vi "Enqueue.vi"(0 "Queue Ref In":refnum<queue>, 5 "State In":string, 11 "error in (no error)":errorcluster) -> (4 "Queue Ref Out":refnum<queue>, 15 "error out":errorcluster)   [LabVIEW 2019, in "Queue Driver.lvlib"]
uses:
  Queue Driver.lvlib
  TypeDefs/Queue Data.ctl
  TypeDefs/Queue Operation.ctl
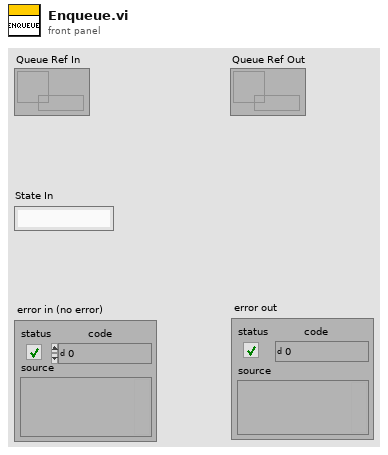
[diagram p1: front panel]
types:
  T1 = typedef "Queue Driver.lvlib/Queue Operation.ctl" = enum16{"Create", "Enqueue", "EnqueueN", "Dequeue", "Flush", "Destroy"}
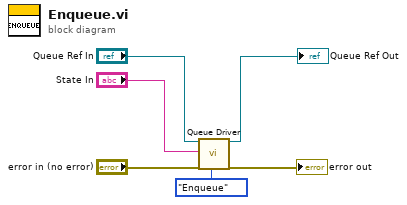
[diagram p0: block diagram]
diagram:
  n1 = call "Queue Driver.vi"("Queue Ref In"="Queue Ref In", "State In"="State In", "error in (no error)"="error in (no error)", "Queue Operation"=Queue_Operation."Enqueue") -> ("Queue Ref Out"=→"Queue Ref Out":refnum<queue>, "error out"=→"error out":errorcluster)  [unwired: 12 in, 2 out]
